vi "PPMSDR_Log_Parse.vi"(11 "file path (dialog if empty)":path=path "\\\\PPMS\\Data/logppmsdata_20160520.dat") -> (2 "Array 2":cluster{timestamp[], dbl[]}[](array[cluster]), 3 "Array":string[](array[string])=["PPMSDR Comment", "PPMSDR Time Stamp (sec)", "PPMSDR Status (code)", "PPMSDR Temperature (K)", "PPMSDR Magnetic Field (Oe)", "PPMSDR Sample Position (deg)", "PPMSDR Bridge 1 Resistance (ohms)", "PPMSDR Bridge 1 Excitation (uA)", "PPMSDR Bridge 2 Resistance (ohms)", "PPMSDR Bridge 2 Excitation (uA)", "PPMSDR Bridge 3 Resistance (ohms)", "PPMSDR Bridge 3 Excitation (uA)", "PPMSDR Bridge 4 Resistance (ohms)", "PPMSDR Bridge 4 Excitation (uA)", "PPMSDR Signal 1 Vin (V)", "PPMSDR Signal 2 Vin (V)", "PPMSDR Digital Inputs (code)", "PPMSDR Drive 1 Iout (mA)", "PPMSDR Drive 1 Ipower (watts)", "PPMSDR Drive 2 Iout (mA)", "PPMSDR Drive 2 Ipower (watts)", "PPMSDR Pressure ()", "PPMSDR Map 20 ()", "PPMSDR Map 21 ()", "PPMSDR Map 22 ()", "PPMSDR Map 23 ()", "PPMSDR Map 24 ()", "PPMSDR Map 25 ()", "PPMSDR Map 26 ()", "PPMSDR Map 27 ()", "PPMSDR Map 28 ()", "PPMSDR Map 29 ()", "PPMSDR System Status (code)", "PPMSDR Setpoint (K)", "PPMSDR Magnet (Oe)", "PPMSDR Valve Position (deg)", "PPMSDR CIG Cernox (K)", "PPMSDR CIG Excit (uA)", "PPMSDR Plat Therm (K)", "PPMSDR Plat Excit (uA)", "PPMSDR Neck Therm (K)", "PPMSDR Neck Excit (uA)", "PPMSDR Spare Therm (K)", "PPMSDR Spare Excit (uA)", "PPMSDR Flow Rate (l min)", "PPMSDR Annulus Vacuum (V)", "PPMSDR Impedance (mode)", "PPMSDR Block Htr Cur (mA)", "PPMSDR Block Htr Pwr (W)", "PPMSDR Neck Htr Cur (mA)", "PPMSDR Neck Htr Pwr (W)", "PPMSDR Annulus Pres (Torr)", "PPMSDR System Pres (Torr)", "PPMSDR Tableless Map53 ()", "PPMSDR Tableless Map54 ()", "PPMSDR Redirected 55 ()", "PPMSDR Redirected 56 ()", "PPMSDR Redirected 57 ()", "PPMSDR Redirected 58 ()", "PPMSDR Redirected 59 ()", "PPMSDR EXT Flow (L min)", "PPMSDR Redirected 61 ()", "PPMSDR Seq Stat ()", "PPMSDR Sys Temp ()", "PPMSDR He Level ()", "PPMSDR Map 67 ()", "PPMSDR Map 68 ()", "PPMSDR Map 69 ()", "PPMSDR low res (A) read", "PPMSDR Hi res (A) read", "PPMSDR Mag (V) read", "PPMSDR Mag adj sc(I)set", "PPMSDR Sw heater state", "PPMSDR DAC  I  (cnts)", "PPMSDR Therm v", "PPMSDR KRPMs", "PPMSDR Pump temp (C)", "PPMSDR Pump power (W)", "PPMSDR High Vacuum mode", "PPMSDR Flapper state", "PPMSDR Regen htr flag", "PPMSDR iso flag", "PPMSDR BlockHeater(Ohm)", "PPMSDR NeckHeater(Ohm)", "PPMSDR Last 2 eng st", "PPMSDR Hires enable", "PPMSDR Mag (V) set", "PPMSDR Map 89 ()", "PPMSDR Map 90 ()", "PPMSDR Map 91 ()", "PPMSDR Map 92 ()", "PPMSDR Map 93 ()", "PPMSDR MAP 1", "PPMSDR MAP 2", "PPMSDR MAP 3", "PPMSDR MAP 4", "PPMSDR MAP 5", "PPMSDR MAP 6", "PPMSDR MAP 7", "PPMSDR MAP 8", "PPMSDR MAP 9", "PPMSDR MAP 10", "PPMSDR MAP 11", "PPMSDR MAP 12", "PPMSDR MAP 13", "PPMSDR MAP 14", "PPMSDR MAP 15", "PPMSDR MAP 16", "PPMSDR MAP 17", "PPMSDR MAP 18", "PPMSDR MAP 19", "PPMSDR MAP 20", "PPMSDR MAP 21", "PPMSDR MAP 22", "PPMSDR MAP 23", "PPMSDR MAP 24", "PPMSDR MAP 25", "PPMSDR MAP 26", "PPMSDR MAP 27", "PPMSDR MAP 28", "PPMSDR MAP 29", "PPMSDR MAP 30"])   [LabVIEW 2016]
uses:
  <vilib>/Utility/file.llb/Read From Spreadsheet File (string).vi
panel:
  out "XY Graph":cluster{timestamp[], dbl[]}(graph)
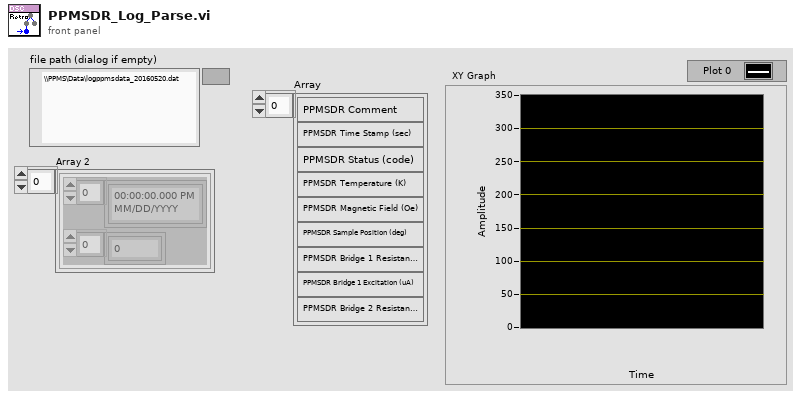
[diagram p1: front panel]
types:
  T1 = cluster{"second":i32, "minute":i32, "hour":i32, "day of month":i32, "month":i32, "year":i32, "day of week":i32, "day of year":i32, "is DST":i32}
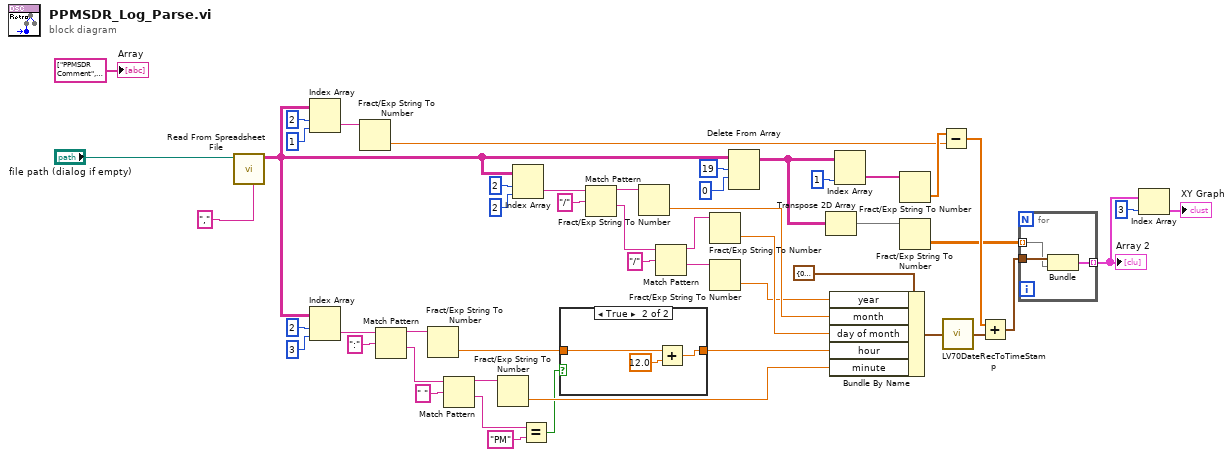
[diagram p0: block diagram]
diagram:
  n1 = call-poly <vilib>:"Read From Spreadsheet File.vi"("delimiter (\\t)"="," ("delimiter (\\t)"), "file path (dialog if empty)"="file path (dialog if empty)") -> ("all rows"=w10:string[][])  [unwired: 5 in, 4 out]
  n2 = Index Array(array=w10, index (row)=2, index (col)=1 ("disabled index (col)")) -> (element=w15:string)
  n3 = Index Array(array=w10, index (row)=2, index (col)=3 ("disabled index (col)")) -> (element=w28:string)
  n4 = Fract/Exp String To Number(string=w15) -> (number=w13:dbl)  [unwired: 3 in, 1 out]
  n5 = Match Pattern(string=w28, regular expression=":" ("search string/char (-)")) -> (before substring=w27:string, after substring=w26:string)  [unwired: 1 in, 2 out]
  n6 = Fract/Exp String To Number(string=w27) -> (number=w19:dbl)  [unwired: 3 in, 1 out]
  n7 = Match Pattern(string=w26, regular expression=" ") -> (before substring=w24:string, after substring=w22:string)  [unwired: 1 in, 2 out]
  n8 = Fract/Exp String To Number(string=w24) -> (number=w23:dbl)  [unwired: 3 in, 1 out]
  n9 = Index Array(array=w10, index (row)=2, index (col)=2 ("disabled index (col)")) -> (element=w41:string)
  n10 = Equal?(x=w22, y="PM") -> (x = y?=w20:bool)
  n11 = case shown="True" w20 {
    tunnel: w19 -> [w51 w54]
    tunnel: [w51 w52] -> w18
    frame False {
    }
    frame True {
      n12 = Add(x=w54, y=12.0) -> (x+y=w52:dbl)
    }
  }
  n13 = Match Pattern(string=w41, regular expression="/" ("search string/char (-)")) -> (before substring=w36:string, after substring=w31:string)  [unwired: 1 in, 2 out]
  n14 = Fract/Exp String To Number(string=w36) -> (number=w35:dbl)  [unwired: 3 in, 1 out]
  n15 = Match Pattern(string=w31, regular expression="/" ("search string/char (-)")) -> (before substring=w34:string, after substring=w30:string)  [unwired: 1 in, 2 out]
  n16 = Fract/Exp String To Number(string=w34) -> (number=w33:dbl)  [unwired: 3 in, 1 out]
  n17 = Fract/Exp String To Number(string=w30) -> (number=w32:dbl)  [unwired: 3 in, 1 out]
  n18 = Delete From Array(array=w10, length=19, index (row)=0) -> (array with subset deleted=w9:string[][])  [unwired: 1 in, 1 out]
  n19 = Transpose 2D Array(2D array=w9) -> (transposed array=w8:string[][])
  n20 = Bundle By Name(cluster=T1 {"second"=0, "minute"=0, "hour"=0, "day of month"=0, "month"=0, "year"=0, "day of week"=0, "day of year"=0, "is DST"=0} ("date time rec"), "year"=w32, "month"=w35, "day of month"=w33, "hour"=w18, "minute"=w23) -> (w38:T1)
  n21 = Index Array(array=w9, index (col)=1 ("disabled index (col)")) -> (element=w48:string[])  [unwired: 1 in]
  n22 = Fract/Exp String To Number(string=w48) -> (number=w14:dbl[])  [unwired: 3 in, 1 out]
  n23 = Fract/Exp String To Number(string=w8) -> (number=w6:dbl[][])  [unwired: 3 in, 1 out]
  n24 = Subtract(x=w14, y=w13) -> (x-y=w11:dbl[])
  n25 = call <vilib>:"LV70DateRecToTimeStamp.vi"("date time rec"=w38) -> ("Time Stamp"=w12:timestamp)
  n26 = Add(x=w11, y=w12) -> (x+y=w7:timestamp[])
  n27 = for {
    tunnel: w7 -> [w57]
    tunnel: w6 -> [w56] mode=indexing
    tunnel: [w55] -> w3 mode=indexing
    n28 = Bundle(w57, w56) -> (w55:cluster{timestamp[], dbl[]})  [unwired: 1 in]
  }
  "Array 2" <- w3
  n29 = Index Array(array=w3, index=3) -> (element=→"XY Graph":cluster{timestamp[], dbl[]})
  "Array" <- string[] ["PPMSDR Comment", "PPMSDR Time Stamp (sec)", "PPMSDR Status (code)", "PPMSDR Temperature (K)", "PPMSDR Magnetic Field (Oe)", "PPMSDR Sample Position (deg)", "PPMSDR Bridge 1 Resistance (ohms)", "PPMSDR Bridge 1 Excitation (uA)", "PPMSDR Bridge 2 Resistance (ohms)", "PPMSDR Bridge 2 Excitation (uA)", "PPMSDR Bridge 3 Resistance (ohms)", "PPMSDR Bridge 3 Excitation (uA)", "PPMSDR Bridge 4 Resistance (ohms)", "PPMSDR Bridge 4 Excitation (uA)", "PPMSDR Signal 1 Vin (V)", "PPMSDR Signal 2 Vin (V)", "PPMSDR Digital Inputs (code)", "PPMSDR Drive 1 Iout (mA)", "PPMSDR Drive 1 Ipower (watts)", "PPMSDR Drive 2 Iout (mA)", "PPMSDR Drive 2 Ipower (watts)", "PPMSDR Pressure ()", "PPMSDR Map 20 ()", "PPMSDR Map 21 ()", "PPMSDR Map 22 ()", "PPMSDR Map 23 ()", "PPMSDR Map 24 ()", "PPMSDR Map 25 ()", "PPMSDR Map 26 ()", "PPMSDR Map 27 ()", "PPMSDR Map 28 ()", "PPMSDR Map 29 ()", "PPMSDR System Status (code)", "PPMSDR Setpoint (K)", "PPMSDR Magnet (Oe)", "PPMSDR Valve Position (deg)", "PPMSDR CIG Cernox (K)", "PPMSDR CIG Excit (uA)", "PPMSDR Plat Therm (K)", "PPMSDR Plat Excit (uA)", "PPMSDR Neck Therm (K)", "PPMSDR Neck Excit (uA)", "PPMSDR Spare Therm (K)", "PPMSDR Spare Excit (uA)", "PPMSDR Flow Rate (l min)", "PPMSDR Annulus Vacuum (V)", "PPMSDR Impedance (mode)", "PPMSDR Block Htr Cur (mA)", "PPMSDR Block Htr Pwr (W)", "PPMSDR Neck Htr Cur (mA)", "PPMSDR Neck Htr Pwr (W)", "PPMSDR Annulus Pres (Torr)", "PPMSDR System Pres (Torr)", "PPMSDR Tableless Map53 ()", "PPMSDR Tableless Map54 ()", "PPMSDR Redirected 55 ()", "PPMSDR Redirected 56 ()", "PPMSDR Redirected 57 ()", "PPMSDR Redirected 58 ()", "PPMSDR Redirected 59 ()", "PPMSDR EXT Flow (L min)", "PPMSDR Redirected 61 ()", "PPMSDR Seq Stat ()", "PPMSDR Sys Temp ()", "PPMSDR He Level ()", "PPMSDR Map 67 ()", "PPMSDR Map 68 ()", "PPMSDR Map 69 ()", "PPMSDR low res (A) read", "PPMSDR Hi res (A) read", "PPMSDR Mag (V) read", "PPMSDR Mag adj sc(I)set", "PPMSDR Sw heater state", "PPMSDR DAC  I  (cnts)", "PPMSDR Therm v", "PPMSDR KRPMs", "PPMSDR Pump temp (C)", "PPMSDR Pump power (W)", "PPMSDR High Vacuum mode", "PPMSDR Flapper state", "PPMSDR Regen htr flag", "PPMSDR iso flag", "PPMSDR BlockHeater(Ohm)", "PPMSDR NeckHeater(Ohm)", "PPMSDR Last 2 eng st", "PPMSDR Hires enable", "PPMSDR Mag (V) set", "PPMSDR Map 89 ()", "PPMSDR Map 90 ()", "PPMSDR Map 91 ()", "PPMSDR Map 92 ()", "PPMSDR Map 93 ()", "PPMSDR MAP 1", "PPMSDR MAP 2", "PPMSDR MAP 3", "PPMSDR MAP 4", "PPMSDR MAP 5", "PPMSDR MAP 6", "PPMSDR MAP 7", "PPMSDR MAP 8", "PPMSDR MAP 9", "PPMSDR MAP 10", "PPMSDR MAP 11", "PPMSDR MAP 12", "PPMSDR MAP 13", "PPMSDR MAP 14", "PPMSDR MAP 15", "PPMSDR MAP 16", "PPMSDR MAP 17", "PPMSDR MAP 18", "PPMSDR MAP 19", "PPMSDR MAP 20", "PPMSDR MAP 21", "PPMSDR MAP 22", "PPMSDR MAP 23", "PPMSDR MAP 24", "PPMSDR MAP 25", "PPMSDR MAP 26", "PPMSDR MAP 27", "PPMSDR MAP 28", "PPMSDR MAP 29", "PPMSDR MAP 30"] ("Array")
